vi "Get Shift.vi"(8 "error in (no error)":errorcluster, 9 "Current Time":timestamp, 10 "Time Stamp Out":timestamp[](array[timestamp])) -> (0 "error out":errorcluster, 2 "Shift":i32)   [LabVIEW 2014]
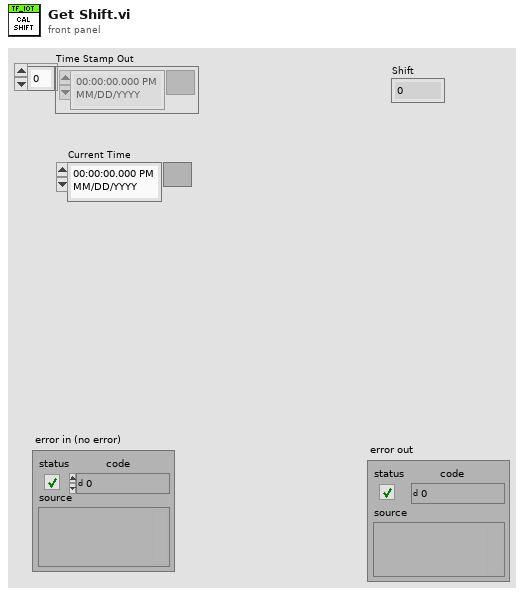
[diagram p1: front panel]
types:
  T1 = typedef "LVDateTimeRec.ctl" = cluster{"fractional second":dbl, "second":i32, "minute":i32, "hour":i32, "day of month":i32, "month":i32, "year":i32, "day of week":i32, "day of year":i32, "DST":i32}
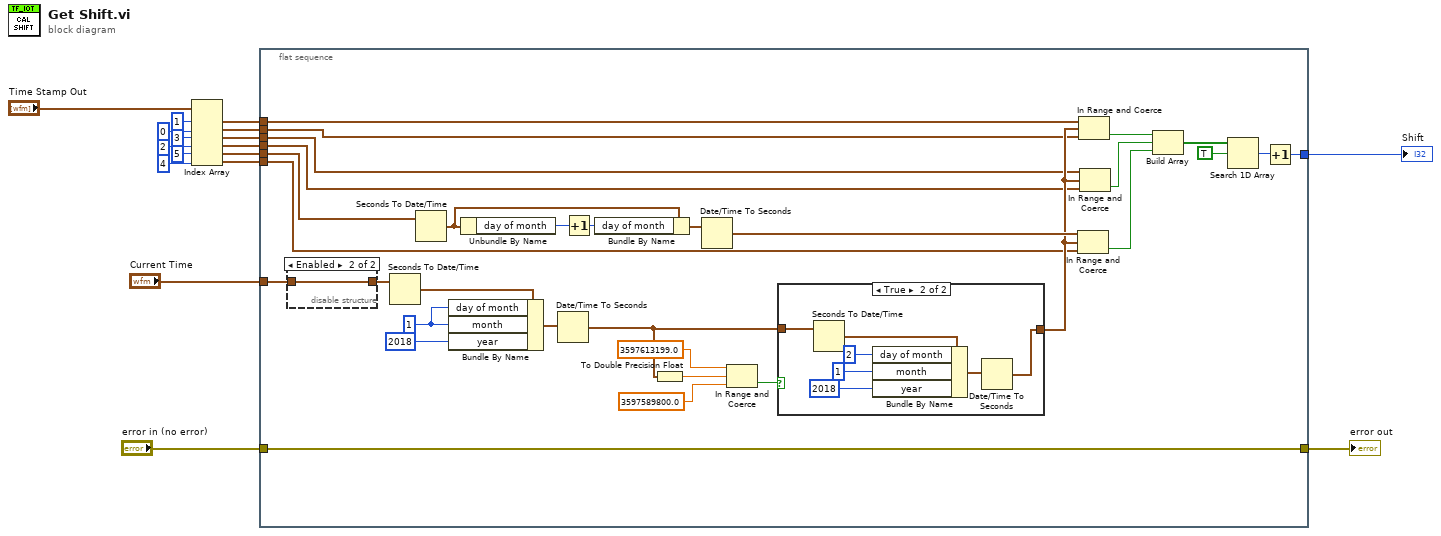
[diagram p0: block diagram]
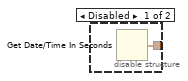
[diagram p2: hidden frame]
diagram:
  n1 = Index Array(array="Time Stamp Out", index #1=1 ("index"), index #2=0 ("index"), index #3=3 ("index"), index #4=2 ("index"), index #5=5 ("index"), index #6=4 ("index")) -> (element #1=w10:timestamp, element #2=w9:timestamp, element #3=w6:timestamp, element #4=w5:timestamp, element #5=w2:timestamp, element #6=w1:timestamp)
  n2 = flat-sequence {
    tunnel: [w37] -> w17
    tunnel: "error in (no error)" -> [w26]
    tunnel: [w26] -> w15
    tunnel: "Current Time" -> [w18]
    tunnel: w10 -> [w25]
    tunnel: w9 -> [w24]
    tunnel: w6 -> [w23]
    tunnel: w5 -> [w22]
    tunnel: w2 -> [w21]
    tunnel: w1 -> [w20]
    frame #0 {
      w30 = 1 ("day of month")
      n3 = disable-structure shown="Enabled" {
        disable-tunnel: [w49 w50] -> w19
        disable-tunnel: w18 -> [_ w50]
        frame Disabled {
          n4 = Get Date/Time In Seconds() -> (seconds since 1Jan1904=w49:timestamp)
        }
        frame Enabled {
        }
      }
      n5 = Seconds To Date/Time(time stamp (now)=w19) -> (date time rec=w34:T1)  [unwired: 1 in]
      n6 = Seconds To Date/Time(time stamp (now)=w21) -> (date time rec=w47:T1)  [unwired: 1 in]
      n7 = Bundle By Name(cluster=w34, "day of month"=w30, "month"=w30, "year"=2018) -> (w36:T1)
      n8 = Unbundle By Name(w47) -> ("day of month"=w45:i32)
      n9 = Date/Time To Seconds(2:w36) -> (0:w28:timestamp)  [unwired: 1 in]
      n10 = Increment(x=w45) -> (x+1=w46:i32)
      n11 = Bundle By Name(cluster=w47, "day of month"=w46) -> (w48:T1)
      n12 = To Double Precision Float(number=w28) -> (double precision float=w31:dbl)
      n13 = Date/Time To Seconds(2:w48) -> (0:w44:timestamp)  [unwired: 1 in]
      n14 = In Range and Coerce(upper limit=3597613199.0 ("double precision float 2"), x=w31, lower limit=3597589800.0 ("double precision float")) -> (In Range?=w29:bool)  [unwired: 1 out]
      n15 = case shown="True" w29 {
        tunnel: w28 -> [w51 w54]
        tunnel: [w51 w53] -> w27
        frame False {
        }
        frame True {
          n16 = Seconds To Date/Time(time stamp (now)=w54) -> (date time rec=w56:T1)  [unwired: 1 in]
          n17 = Bundle By Name(cluster=w56, "day of month"=2, "month"=1 ("day of month"), "year"=2018) -> (w58:T1)
          n18 = Date/Time To Seconds(2:w58) -> (0:w53:timestamp)  [unwired: 1 in]
        }
      }
      n19 = In Range and Coerce(upper limit=w44, x=w27, lower limit=w20) -> (In Range?=w41:bool)  [unwired: 1 out]
      n20 = In Range and Coerce(upper limit=w25, x=w27, lower limit=w24) -> (In Range?=w43:bool)  [unwired: 1 out]
      n21 = In Range and Coerce(upper limit=w23, x=w27, lower limit=w22) -> (In Range?=w42:bool)  [unwired: 1 out]
      n22 = Build Array(w43, w42, w41) -> (w40:bool[])
      n23 = Search 1D Array(1D array=w40, element=TRUE) -> (index of element=w38:i32)  [unwired: 1 in]
      n24 = Increment(x=w38) -> (x+1=w37:i32)
    }
  }
  "Shift" <- w17
  "error out" <- w15
